vi "Actor Core.vi"(8 "error in":errorcluster, 11 "MainWindow in":refnum<class "MainWindow.lvclass">) -> (0 "error out":errorcluster, 3 "Actor out":refnum<class "Actor.lvclass">)   [LabVIEW 2020, in "MainWindow.lvlib" / "MainWindow.lvclass"]
doc: "(<B>Filename</B>: Actor Framework.lvlib:Actor.lvclass:Actor Core.vi)\n\nReceives messages to the actor, reacts to them, and initiates any error handling that may shut the actor down.\n\nDescendant classes may override this VI to append parallel tasks for the actor to complete while it handles messages. Overrides use the Call Parent Class Method node."
uses:
  MainWindow.lvclass
  C:/Program Files (x86)/National Instruments/LabVIEW 2020/vi.lib/MGI/Panel Manager/Panel Actor/Panel Actor/Panel Actor.lvclass
  C:/Program Files (x86)/National Instruments/LabVIEW 2020/vi.lib/ActorFramework/Actor/Actor.lvclass
  <vilib>/ActorFramework/Actor/Actor.lvclass
  Menu/Menu/Menu.lvclass
  Page/Page/Page.lvclass
  MainWindow.lvclass/MainWindow.ctl
  <vilib>/ActorFramework/Message Enqueuer/Message Enqueuer.lvclass/Message Enqueuer.ctl
  <vilib>/ActorFramework/Message Enqueuer/Enqueue.vi
  <vilib>/MGI/Panel Manager/Panel/Panel/Subpanel/Subpanel.lvclass
  C:/Program Files (x86)/National Instruments/LabVIEW 2020/vi.lib/MGI/Panel Manager/Panel/Panel/Panel.lvclass
  <vilib>/ActorFramework/Stop Msg/Stop Msg.lvclass
  C:/Program Files (x86)/National Instruments/LabVIEW 2020/vi.lib/ActorFramework/Message/Message.lvclass
  <vilib>/ActorFramework/Message Priority Queue/Priority Enqueue.vi
  <vilib>/MGI/Panel Manager/Panel Actor/Panel Actor/Panel Actor.lvclass
  <vilib>/MGI/Panel Manager/Panel/Panel/Subpanel/Subpanel.vi
  <vilib>/MGI/Panel Manager/Panel/Panel.lvlib
  C:/Program Files (x86)/National Instruments/LabVIEW 2020/vi.lib/MGI/Monitored Actor/Monitored Actor/Monitored Actor/Monitored Actor.lvclass
  C:/Users/Test/Desktop/MGIPanelActor-Exploration/MainWindow/MainWindow/MainWindow.lvclass
  C:/Program Files (x86)/National Instruments/LabVIEW 2020/vi.lib/MGI/Panel Manager/Panel/Panel/Subpanel/Subpanel.lvclass
  C:/Users/Test/Desktop/MGIPanelActor-Exploration/Menu/Menu/Menu.lvclass
  C:/Users/Test/Desktop/MGIPanelActor-Exploration/Page/Page/Page.lvclass
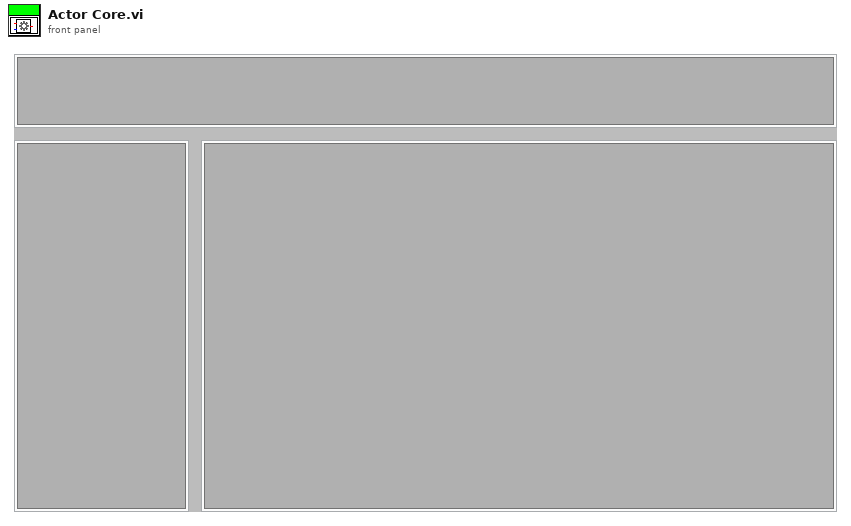
[diagram p1: front panel]
types:
  T1 = map{string, refnum<class "Message Enqueuer.lvclass">}
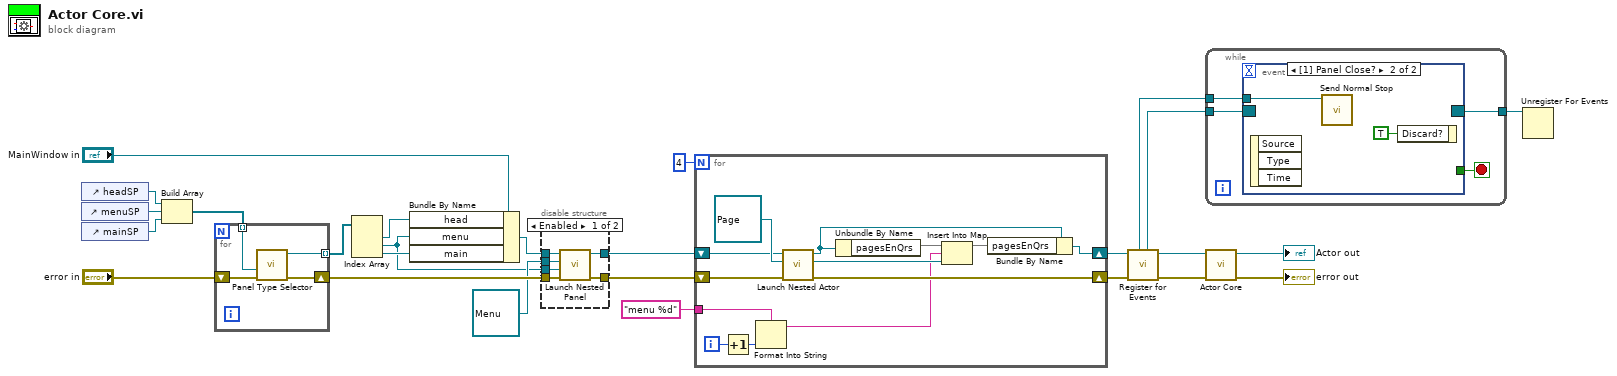
[diagram p0: block diagram]
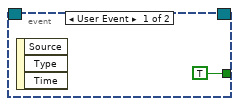
[diagram p3: hidden frame]
diagram:
  n1 = control-ref of="headSP"() -> (w22:refnum<vi>)
  n2 = control-ref of="menuSP"() -> (w16:refnum<vi>)
  n3 = control-ref of="mainSP"() -> (w15:refnum<vi>)
  n4 = Build Array(w22, w16, w15) -> (w21:refnum<vi>[])
  n5 = for {
    tunnel: w21 -> [w30] mode=indexing
    tunnel: [w29] -> w20 mode=indexing
    shift-right: [w27] -> w18
    shift-left: "error in" -> [w28]
    n6 = call-poly <vilib>:"Panel Type Selector.vi"("Error In"=w28, "Sub Panel"=w30) -> ("Error Out"=w27:errorcluster, "Subpanel Out"=w29:refnum<class "Subpanel.lvclass">)  [unwired: 8 in]
  }
  n7 = Index Array(array=w20) -> (element #1=w14:refnum<class "Subpanel.lvclass">, element #2=w7:refnum<class "Subpanel.lvclass">, element #3=w13:refnum<class "Subpanel.lvclass">)  [unwired: 3 in]
  n8 = Bundle By Name(cluster="MainWindow in", "head"=w14, "menu"=w7, "main"=w13) -> (w12:refnum<class "MainWindow.lvclass">)
  n9 = disable-structure shown="Enabled" {
    disable-tunnel: [w36 w38] -> w3
    disable-tunnel: [w35 w37] -> w6
    disable-tunnel: w18 -> [w34 w37]
    disable-tunnel: w12 -> [w33 w38]
    disable-tunnel: refnum<class "Menu.lvclass"> refnum ("Menu.lvlib:Menu.lvclass") -> [w32 _]
    disable-tunnel: w7 -> [w31 _]
    frame Enabled {
      n10 = call <vilib>:"Launch Nested Panel.vi"("error in (no error)"=w34, "Panel"=w31, "Nested Panel Actor"=w32, "Panel Actor in"=w33) -> ("error out"=w35:errorcluster, "Panel Actor out"=w36:refnum<class "MainWindow.lvclass">)  [unwired: 4 in, 2 out]
    }
    frame Disabled {
    }
  }
  n11 = for {
    N: 4 -> [_]
    tunnel: "menu %d" ("Debug Alias") -> [w41]
    shift-right: [w50] -> w5
    shift-left: w6 -> [w51]
    shift-right: [w48] -> w4
    shift-left: w3 -> [w47]
    i -> [w40]
    n12 = Increment(x=w40) -> (x+1=w39:i32)
    n13 = Format Into String(format string=w41, w39) -> (resulting string=w42:string)  [unwired: 2 in, 1 out]
    n14 = call <vilib>:"Launch Nested Actor.vi"("error in (no error)"=w51, "Nested Actor"=refnum<class "Page.lvclass"> refnum ("Page.lvlib:Page.lvclass"), "Caller Actor in"=w47) -> ("error out"=w50:errorcluster, "Nested Actor's Enqueuer"=w44:refnum<class "Message Enqueuer.lvclass">, "Caller Actor out"=w43:refnum<class "MainWindow.lvclass">)  [unwired: 6 in]
    n15 = Unbundle By Name(w43) -> ("pagesEnQrs"=w46:T1)
    n16 = Insert Into Map(map in=w46, key=w42, value=w44) -> (map out=w45:T1)  [unwired: 2 out]
    n17 = Bundle By Name(cluster=w43, "pagesEnQrs"=w45) -> (w48:refnum<class "MainWindow.lvclass">)
  }
  n18 = call <vilib>:"Register for Events.vi"("Error In"=w5, "Panel Actor in"=w4) -> ("Error Out"=w23:errorcluster, "Panel Actor out"=w24:refnum<class "MainWindow.lvclass">, "Pnl Actor"=w11:refnum<event-registration>, "Self Enqueuer"=w9:refnum<class "Message Enqueuer.lvclass">)  [unwired: 6 in]
  n19 = while {
    tunnel: w11 -> [w55]
    tunnel: [w54] -> w10
    tunnel: w9 -> [w53]
    stop <- w52 stop-if-true
    n20 = event shown="[1] Panel Close?" {
      selector: w55 -> [_ _]
      dyn-events: [_ _] -> w54
      timeout: _ -> [_ _]
      tunnel: w53 -> [_ w58]
      tunnel: [TRUE _] -> w52
      event User Event {
        n21 = event-data() -> ()  [unwired: 1 in, 3 out]
      }
      event Panel Close? {
        n22 = event-data() -> ()  [unwired: 1 in, 3 out]
        n23 = call <vilib>:"Send Normal Stop.vi"("Message Enqueuer"=w58) -> ()  [unwired: 10 in, 1 out]
        n24 = event-data("Discard?"=TRUE) -> ()  [unwired: 1 in, 1 out]
      }
    }
  }
  n25 = call-parent "Actor Core.vi"("error in"=w23, "Panel Actor in"=w24) -> ("error out"=→"error out":errorcluster, "Actor out"=→"Actor out":refnum<class "Actor.lvclass">)  [unwired: 8 in]
  n26 = Unregister For Events(event registration refnum=w10) -> ()  [unwired: 1 in, 1 out]
